vi "UP-COUNTER-V1.0.vi"(11 "UPPER LIMIT":u32=30) -> (3 "COUNT":u32)   [LabVIEW 2016]
panel:
  in  "LOWER LIMIT":u32
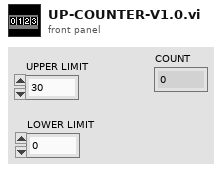
[diagram p1: front panel]
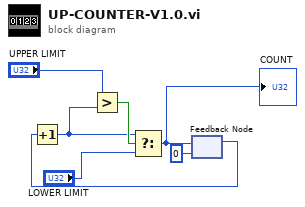
[diagram p0: block diagram]
diagram:
  n1 = feedback #1(u32 0 ("LOWER LIMIT")) -> (w4:u32)
  n2 = Increment(x=w4) -> (x+1=w3:u32)
  n3 = Greater?(x="UPPER LIMIT", y=w3) -> (0:w6:bool)
  n4 = Select(t=w3, s=w6, f="LOWER LIMIT") -> (s? t:f=w2:u32)
  "COUNT" <- w2
  n5 = feedback-in #1(w2) -> ()
